vi "ConfigureChannels.vi"(8 "error in (no error)":errorcluster, 11 "IVI_Class in":refnum<class "IVI_Class.lvclass">) -> (0 "error out":errorcluster, 3 "IVI_Class out":refnum<class "IVI_Class.lvclass">)   [LabVIEW 2014, in "ScopePlugins.lvlib" / "IVI_Class.lvclass"]
uses:
  IVI_Class.lvclass
  ScopePluginBaseClass/ScopePluginsBase.lvclass/ScopePluginsBase.ctl
  ScopePluginBaseClass/Accessors/Read Handle.vi
  ScopePluginBaseClass/Accessors/Read Channels.vi
  ScopePluginBaseClass/Accessors/Read Connected.vi
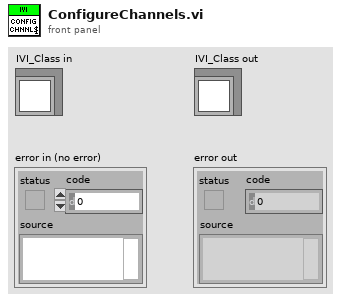
[diagram p1: front panel]
types:
  T1 = typedef "ScopePlugins.lvlib/Channels.ctl" = cluster{"Count":i32, "ChannelArray":T2[]}
  T2 = typedef "ScopePlugins.lvlib/Channel.ctl" = cluster{"Enabled":bool, "Name":string, "InputImpedance":dbl, "InputFreqMax":dbl, "ProbeAttn":dbl, "Coupling":enum16{"AC", "DC", "GND"}, "Offset":dbl, "Range":dbl}
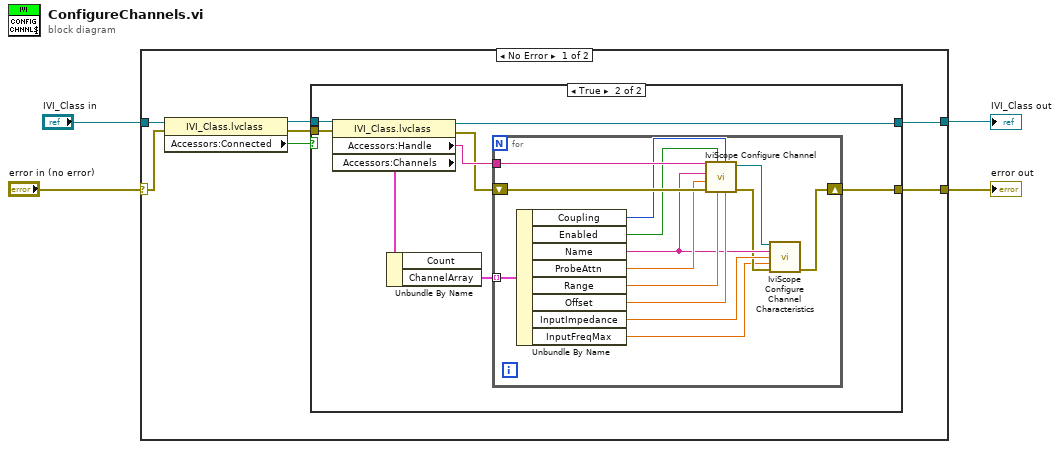
[diagram p0: block diagram]
diagram:
  n1 = case shown="No Error" "error in (no error)" {
    selector: "error in (no error)" -> [w10 w36]
    tunnel: [w7 w37] -> w2
    tunnel: "IVI_Class in" -> [w11 w37]
    tunnel: [w5 w36] -> w1
    frame No Error {
      n2 = property class="IVI_Class.lvclass"(reference=w11, error in=w10) -> (reference out=w8:refnum<class "IVI_Class.lvclass">, error out=w6:errorcluster, "Accessors:Connected"=w9:bool)
      n3 = case shown="True" w9 {
        tunnel: [w13 w14] -> w7
        tunnel: w8 -> [w13 w21]
        tunnel: w6 -> [w12 w20]
        tunnel: [w12 w15] -> w5
        frame False {
        }
        frame True {
          n4 = property class="IVI_Class.lvclass"(reference=w21, error in=w20) -> (reference out=w14:refnum<class "IVI_Class.lvclass">, error out=w16:errorcluster, "Accessors:Handle"=w17:string, "Accessors:Channels"=w19:T1)
          n5 = Unbundle By Name(w19) -> ("ChannelArray"=w18:T2[])  [unwired: 1 out]
          n6 = for {
            tunnel: w18 -> [w35] mode=indexing
            tunnel: w17 -> [w34]
            shift-right: [w22] -> w15
            shift-left: w16 -> [w33]
            n7 = Unbundle By Name(w35) -> ("Coupling"=w32:enum16{"AC", "DC", "GND"}, "Enabled"=w31:bool, "Name"=w26:string, "ProbeAttn"=w30:dbl, "Range"=w29:dbl, "Offset"=w28:dbl, "InputImpedance"=w27:dbl, "InputFreqMax"=w23:dbl)
            n8 = call <vilib>:"IviScope Configure Channel.vi"("vertical offset (0.0 V)"=w28, "vertical coupling (DC)"=w32, "vertical range (10.0 V)"=w29, "channel enabled (True)"=w31, "error in (no error)"=w33, "probe attenuation (1:1.0)"=w30, "channel name (\"CHANNEL1\")"=w26, "instrument handle"=w34) -> ("error out"=w24:errorcluster, "instrument handle out"=w25:refnum<k15>)  [unwired: 2 in]
            n9 = call <vilib>:"IviScope Configure Channel Characteristics.vi"("instrument handle"=w25, "channel name (\"CHANNEL1\")"=w26, "input impedance (1.0E+6 ohms)"=w27, "max input frequency (1.0E+6 Hz)"=w23, "error in (no error)"=w24) -> ("error out"=w22:errorcluster)  [unwired: 9 in, 1 out]
          }
        }
      }
    }
    frame Error {
    }
  }
  "error out" <- w1
  "IVI_Class out" <- w2
